vi "Set Source Destination.vi"(7 "Source Index":i32, 8 "error in (no error)":errorcluster, 10 "Destination Label":string, 11 "BuildSpec in":refnum<vi>) -> (0 "error out":errorcluster, 3 "BuildSpec out":refnum<vi>)   [LabVIEW 2019, in "Project Sync Tools.lvclass"]
uses:
  Project Sync Tools.lvclass
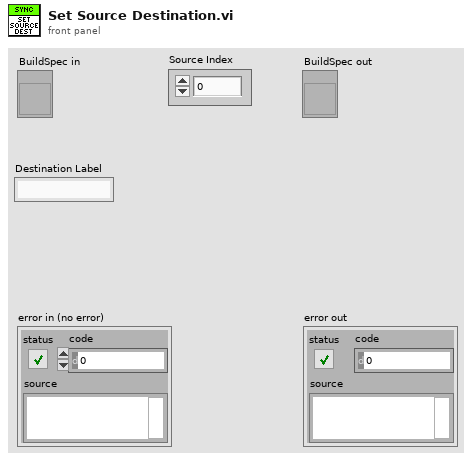
[diagram p1: front panel]
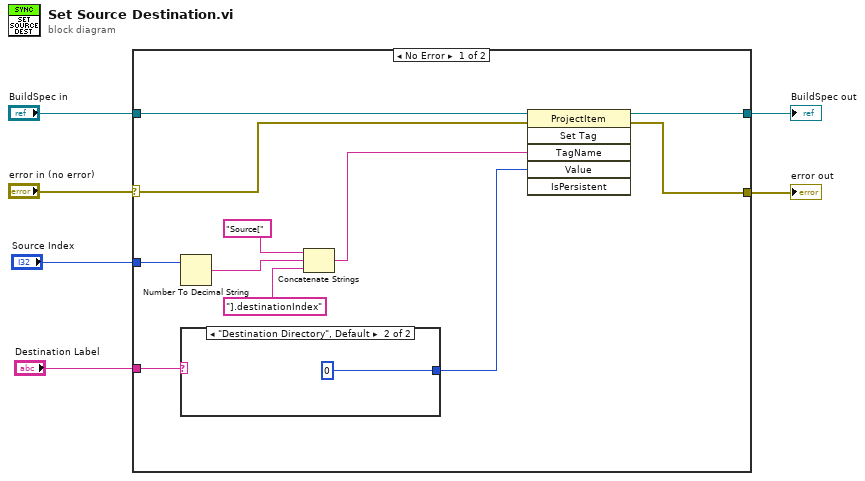
[diagram p0: block diagram]
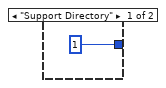
[diagram p2: hidden frame]
diagram:
  n1 = case shown="No Error" "error in (no error)" {
    selector: "error in (no error)" -> [w7 w21]
    tunnel: "BuildSpec in" -> [w17 w20]
    tunnel: [w16 w21] -> w5
    tunnel: [w15 w20] -> w4
    tunnel: "Source Index" -> [w14 _]
    tunnel: "Destination Label" -> [w9 _]
    frame No Error {
      n2 = Number To Decimal String(number=w14) -> (decimal integer string=w12:string)  [unwired: 1 in]
      n3 = case shown="\"Destination Directory\", Default" w9 {
        tunnel: [1 0] -> w8
        frame "Support Directory" {
        }
        frame "Destination Directory", Default {
        }
      }
      n4 = Concatenate Strings("Source[" ("string"), w12, "].destinationIndex") -> (w10:string)
      n5 = invoke class="ProjectItem" method="Set Tag"(reference=w17, error in=w7, "TagName"=w10, "Value"=w8) -> (reference out=w15:refnum<vi>, error out=w16:errorcluster)  [unwired: 2 in, 4 out]
    }
    frame Error {
    }
  }
  "error out" <- w5
  "BuildSpec out" <- w4
